vi "r_dot_decay.vi"(11 "r array in":dbl[](array[numeric])) -> (3 "r dot out":dbl[](array[numeric]))   [LabVIEW 2018]
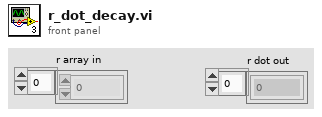
[diagram p1: front panel]
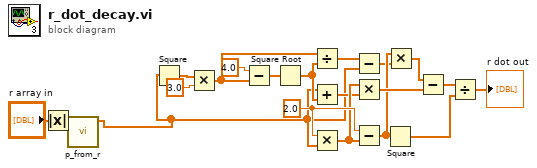
[diagram p0: block diagram]
diagram:
  w15 = 2.0
  n1 = Absolute Value(x="r array in") -> (abs(x)=w1:dbl[])
  n2 = call "p_from_r.vi"("r array in"=w1) -> ("P eff. out"=w2:dbl[])  [unwired: 10 in]
  n3 = Square(x=w2) -> (x^2=w18:dbl[])
  n4 = Multiply(x=w18, y=3.0) -> (x*y=w8:dbl[])
  n5 = Subtract(x=4.0, y=w8) -> (x-y=w16:dbl[])
  n6 = Square Root(x=w16) -> (sqrt(x)=w4:dbl[])
  n7 = Divide(x=w8, y=w4) -> (x/y=w9:dbl[])
  n8 = Add(x=w2, y=w4) -> (x+y=w5:dbl[])
  n9 = Multiply(x=w15, y=w2) -> (x*y=w6:dbl[])
  n10 = Subtract(x=w9, y=w2) -> (x-y=w7:dbl[])
  n11 = Multiply(x=w6, y=w5) -> (x*y=w14:dbl[])
  n12 = Subtract(x=w15, y=w6) -> (x-y=w10:dbl[])
  n13 = Square(x=w10) -> (x^2=w11:dbl[])
  n14 = Multiply(x=w10, y=w7) -> (x*y=w13:dbl[])
  n15 = Subtract(x=w13, y=w14) -> (x-y=w12:dbl[])
  n16 = Divide(x=w12, y=w11) -> (x/y=→"r dot out":dbl[])
